vi "Polar Accumulated Correlation.vi"(4 "Microphone Coordinates (cm, rad)":cluster{"r":dbl, "theta":dbl}[](array[cluster]), 5 "Ntheta":i32=16, 6 "Radius (cm)":dbl=123.4 format="%#_13g", 7 "Nr":i32=16, 8 "Sound Velocity (cm/s)":dbl=576000.0, 9 "Sampling Rate":i32=500000, 11 "Waveforms":dbl[][](array[numeric])) -> (2 "Source Coordinates (cm, rad)":cluster{"r":dbl, "theta":dbl})   [LabVIEW 2013]
uses:
  <vilib>/Analysis/2dsp.llb/1D Cross Correlation (DBL).vi
  <vilib>/Analysis/NI_AALPro.lvlib
panel:
  out "Cross Corr.\n1/2 Length":i32
  out "dTheta":dbl
  out "dR":dbl
  out "Signals":dbl[][](graph)
  out "output variable 3":dbl
  out "output variable 2":dbl
  out "output variable":dbl
  out "subarray":dbl[][](array[numeric])
  out "size(s)":i32[](array[numeric])
  out "Correlation":dbl[][](graph)
  out "Lag Matrix":dbl[][](array[numeric])
  # "Inputs and Outputs"
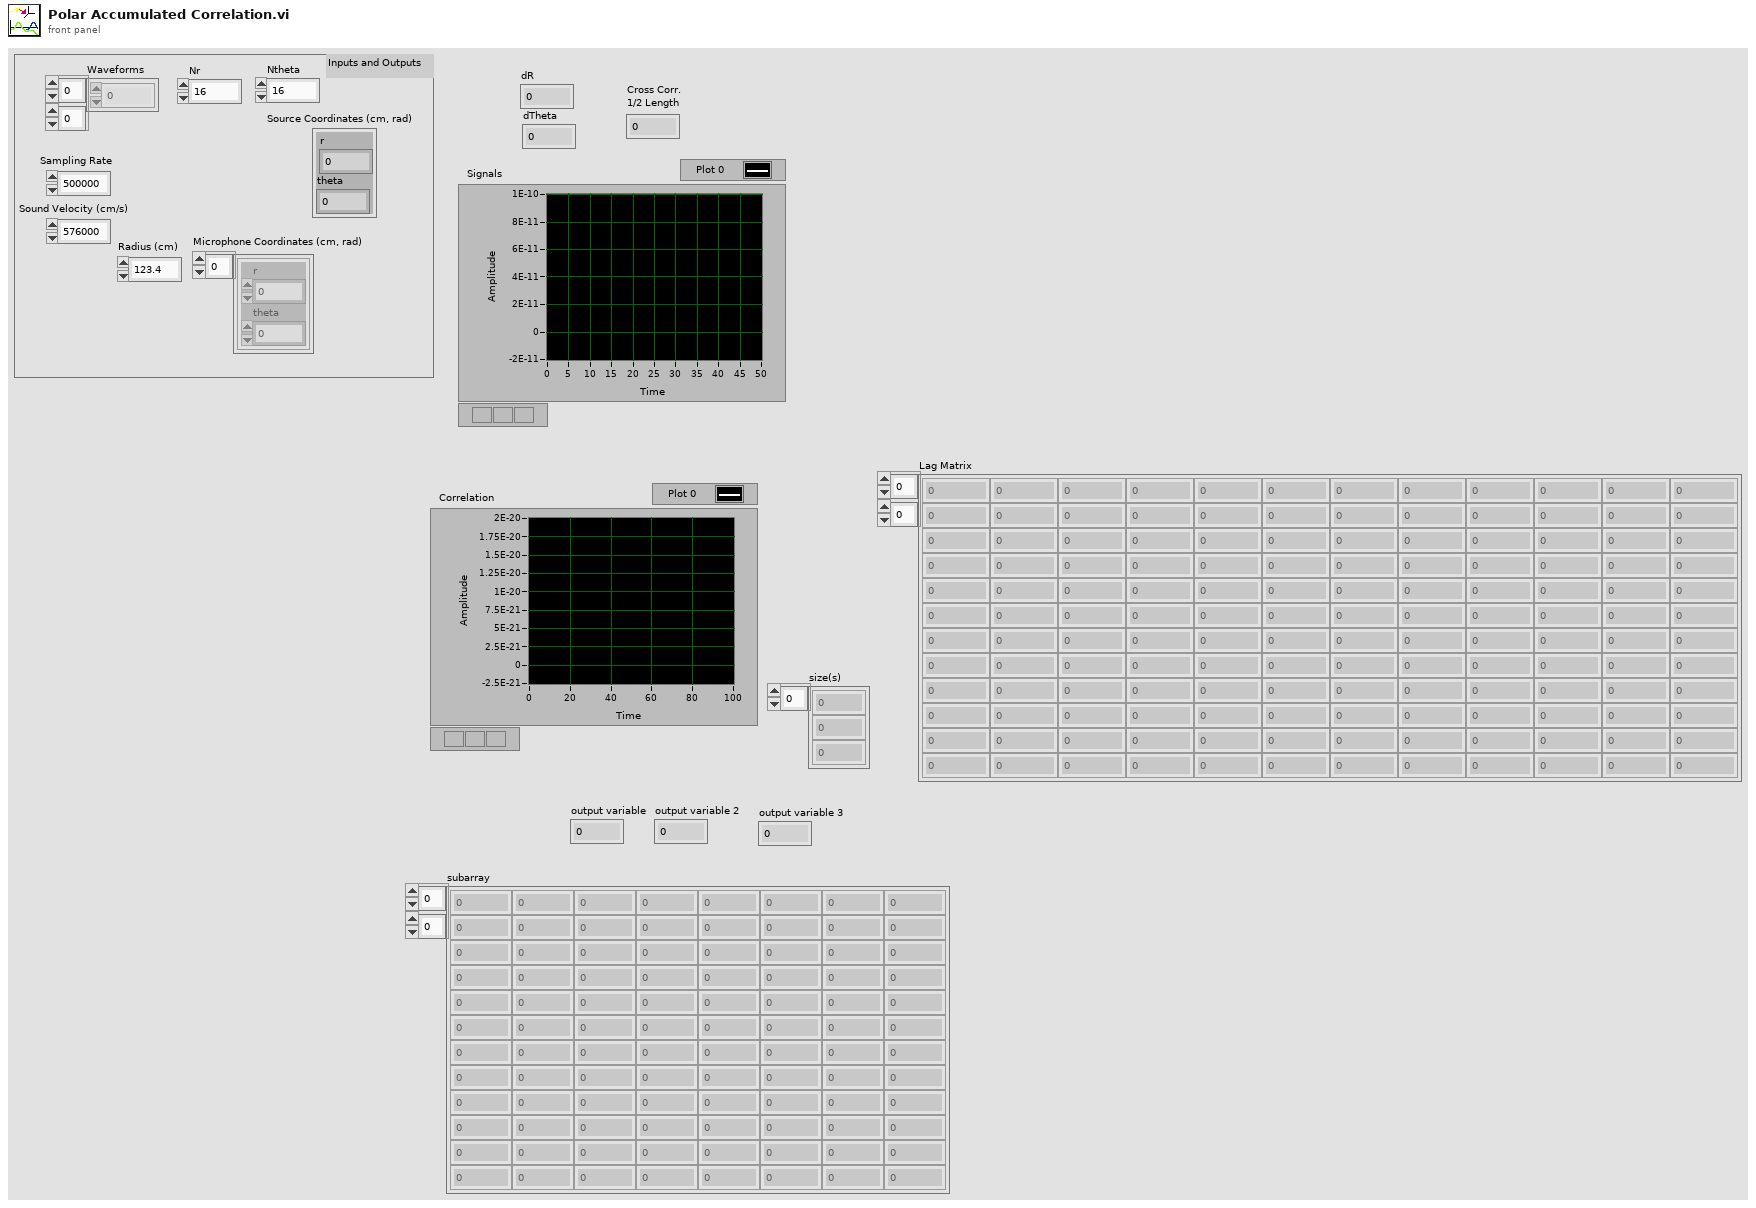
[diagram p1: front panel]
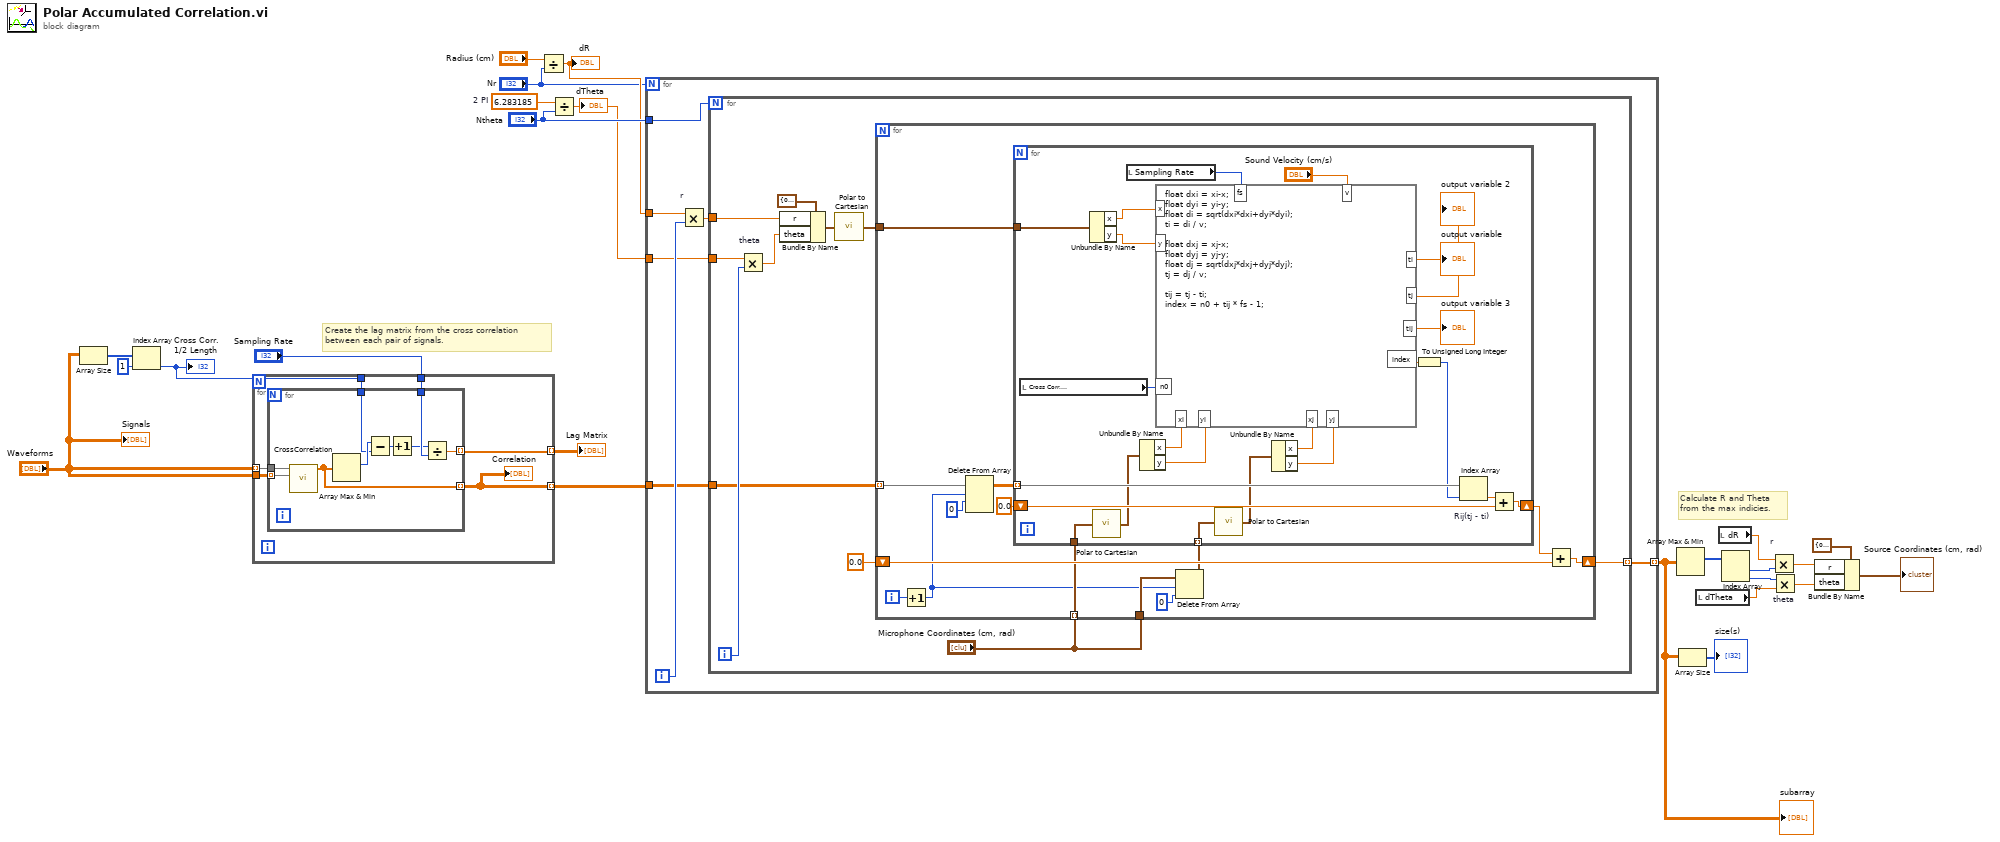
[diagram p0: block diagram]
diagram:
  w22 = 6.283185  # 2 PI
  # "Create the lag matrix from the cross correlation\nbetween each pair of signals."
  # "Calculate R and Theta\nfrom the max indicies."
  n1 = Array Size ("Size(s)")(array="Waveforms") -> (size(s)=w4:i32[])
  n2 = Index Array(array=w4, index=1) -> (element=w2:i32)
  "Cross Corr.\n1/2 Length" <- w2
  n3 = for {
    tunnel: "Waveforms" -> [w26] mode=indexing
    tunnel: "Waveforms" -> [w30]
    tunnel: "Sampling Rate" -> [w29]
    tunnel: [w28] -> w24 mode=indexing
    tunnel: [w27] -> w20 mode=indexing
    tunnel: w2 -> [w25]
    n4 = for {
      tunnel: w30 -> [w39] mode=indexing
      tunnel: w26 -> [w38]
      tunnel: w29 -> [w37]
      tunnel: [w36] -> w28 mode=indexing
      tunnel: [w33] -> w27 mode=indexing
      tunnel: w25 -> [w31]
      n5 = call-poly <vilib>:"CrossCorrelation.vi"("Y"=w39, "X"=w38) -> ("Rxy"=w33:dbl[])  [unwired: 8 in, 1 out]
      n6 = Array Max & Min(array=w33) -> (max index (indices)=w32:i32)  [unwired: 3 out]
      n7 = Subtract(x=w32, y=w31) -> (x-y=w35:i32)
      n8 = Increment(x=w35) -> (x+1=w34:i32)
      n9 = Divide(x=w34, y=w37) -> (x/y=w36:dbl)
    }
    "Correlation" <- w27
  }
  "Lag Matrix" <- w24
  n10 = Divide(x="Radius (cm)", y="Nr") -> (x/y=w17:dbl)
  "dR" <- w17
  n11 = Divide(x=w22, y="Ntheta") -> (x/y=w16:dbl)
  "dTheta" <- w16
  n12 = for {
    N: "Nr" -> [_]
    tunnel: [w46] -> w13 mode=indexing
    tunnel: "Ntheta" -> [w45]
    tunnel: w17 -> [w44]
    tunnel: w16 -> [w42]
    tunnel: w20 -> [w41]
    i -> [w43]
    n13 = Multiply "r"(x=w44, y=w43) -> (x*y=w40:dbl)
    n14 = for {
      N: w45 -> [_]
      tunnel: [w56] -> w46 mode=indexing
      tunnel: w42 -> [w55]
      tunnel: w40 -> [w50]
      tunnel: w41 -> [w53]
      i -> [w54]
      n15 = Multiply "theta"(x=w55, y=w54) -> (x*y=w49:dbl)
      n16 = Bundle By Name(cluster=cluster{"r":dbl, "theta":dbl} {"r"=0.0, "theta"=0.0} ("Polar\nCoordinates"), "r"=w50, "theta"=w49) -> (w47:cluster{"r":dbl, "theta":dbl})
      n17 = call "Polar to Cartesian.vi"("Polar\nCoordinates"=w47) -> ("Cartesian\nCoordinates"=w48:cluster{"x":dbl, "y":dbl})  [unwired: 4 in]
      n18 = for {
        shift-right: [w69] -> w56
        shift-left: 0.0 -> [w70]
        tunnel: "Microphone Coordinates (cm, rad)" -> [w68] mode=indexing
        tunnel: "Microphone Coordinates (cm, rad)" -> [w66]
        tunnel: w53 -> [w63] mode=indexing
        tunnel: w48 -> [w59]
        i -> [w67]
        n19 = Increment(x=w67) -> (x+1=w60:i32)
        n20 = Delete From Array(array=w63, length=w60, index (row)=0) -> (array with subset deleted=w62:dbl[][])  [unwired: 1 in, 1 out]
        n21 = Delete From Array(array=w66, length=w60, index=0 ("index (row)")) -> (array with subset deleted=w64:cluster{"r":dbl, "theta":dbl}[])  [unwired: 1 out]
        n22 = for {
          shift-right: [w91] -> w71
          shift-left: 0.0 -> [w89]
          tunnel: w64 -> [w76] mode=indexing
          tunnel: w68 -> [w80]
          tunnel: w62 -> [w93] mode=indexing
          tunnel: w59 -> [w83]
          n23 = local read "Cross Corr.\n1/2 Length"() -> (w72:i32)
          n24 = Unbundle By Name(w83) -> ("x"=w82:dbl, "y"=w81:dbl)
          n25 = call "Polar to Cartesian.vi"("Polar\nCoordinates"=w80) -> ("Cartesian\nCoordinates"=w79:cluster{"x":dbl, "y":dbl})  [unwired: 4 in]
          n26 = local read "Sampling Rate"() -> (w85:i32)
          n27 = Unbundle By Name(w79) -> ("x"=w78:dbl, "y"=w77:dbl)
          n28 = call "Polar to Cartesian.vi"("Polar\nCoordinates"=w76) -> ("Cartesian\nCoordinates"=w75:cluster{"x":dbl, "y":dbl})  [unwired: 4 in]
          n29 = Unbundle By Name(w75) -> ("x"=w74:dbl, "y"=w73:dbl)
          n30 = formula code="float dxi = xi-x;\nfloat dyi = yi-y;\nfloat di = sqrt(dxi*dxi+dyi*dyi);\nti = di / v;\n\nfloat dxj = xj-x;\nfloat dyj = yj-y;\nfloat dj = sqrt(dxj*dxj+dyj*dyj);\ntj = dj / v;\n\ntij = tj - ti;\nindex = n0 + tij * fs - 1;"("xi"=w78, "yi"=w77, "xj"=w74, "yj"=w73, "x"=w82, "y"=w81, "v"="Sound Velocity (cm/s)", "fs"=w85, "n0"=w72) -> ("index"=w94:dbl, "ti"=→"output variable":dbl, "tj"=→"output variable 2":dbl, "tij"=→"output variable 3":dbl)
          n31 = To Unsigned Long Integer(number=w94) -> (unsigned 32bit integer=w92:u32)
          n32 = Index Array "Rij(tj - ti)"(array=w93, index=w92) -> (element=w90:dbl)
          n33 = Add(x=w90, y=w89) -> (x+y=w91:dbl)
        }
        n34 = Add(x=w71, y=w70) -> (x+y=w69:dbl)
      }
    }
  }
  "subarray" <- w13
  n35 = Array Max & Min(array=w13) -> (max index (indices)=w19:i32[])  [unwired: 3 out]
  n36 = Array Size(array=w13) -> (size(s)=→"size(s)":i32[])
  n37 = local read "dTheta"() -> (w12:dbl)
  n38 = local read "dR"() -> (w10:dbl)
  n39 = Index Array(array=w19) -> (element #1=w11:i32, element #2=w18:i32)  [unwired: 2 in]
  n40 = Multiply "r"(x=w10, y=w11) -> (x*y=w7:dbl)
  n41 = Multiply "theta"(x=w18, y=w12) -> (x*y=w6:dbl)
  n42 = Bundle By Name(cluster=cluster{"r":dbl, "theta":dbl} {"r"=0.0, "theta"=0.0} ("Polar\nCoordinates"), "r"=w7, "theta"=w6) -> (→"Source Coordinates (cm, rad)":cluster{"r":dbl, "theta":dbl})
  "Signals" <- "Waveforms"
